vi "SID_filter_V2.vi"(5 "sampling info":cluster{"Fs":dbl, "#s":i32}={"Fs"=44100.0, "#s"=50}, 6 "reset":bool, 7 "filter":T1={"freq"=70.6, "res"=240.0, "HP"=FALSE, "BP"=FALSE, "LP"=TRUE, "VC1"=TRUE, "VC2"=TRUE, "VC3"=TRUE, "vol"=1.0} {"vol" format="%0.2f"; "res" format="%0.2f"; "freq" format="%0.2f"}, 9 "VC3":dbl[](array[numeric]), 10 "VC2":dbl[](array[numeric]), 11 "VC1":dbl[](array[numeric])) -> (3 "out":dbl[](array[numeric]))   [LabVIEW 2018]
uses:
  SID_filter_reg.ctl
panel:
  out "R":dbl
  out "Q":dbl
  out "g":dbl
  out "freq":dbl
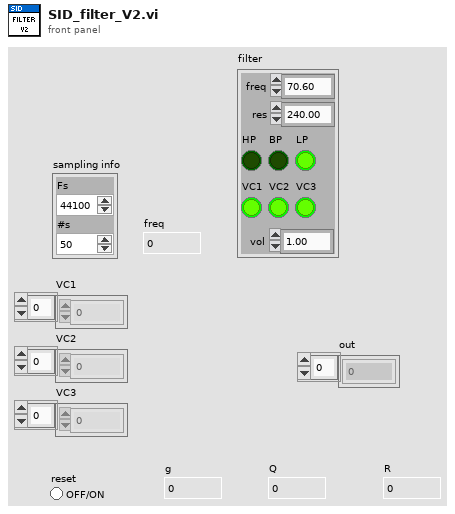
[diagram p1: front panel]
types:
  T1 = typedef "SID_filter_reg.ctl" = cluster{"freq":dbl, "res":dbl, "HP":bool, "BP":bool, "LP":bool, "VC1":bool, "VC2":bool, "VC3":bool, "vol":dbl}
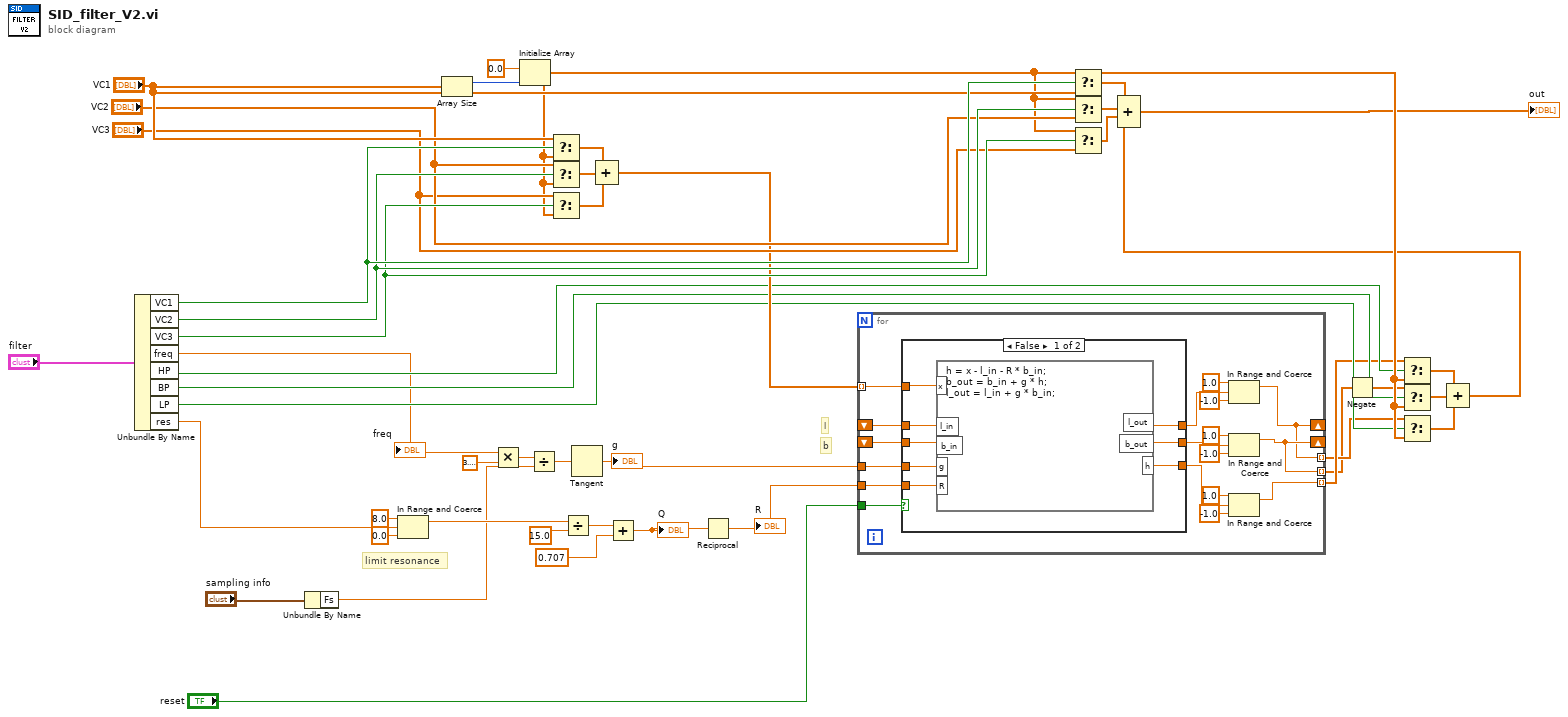
[diagram p0: block diagram]
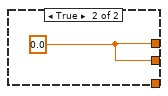
[diagram p2: hidden frame]
diagram:
  # "limit resonance"
  # "b"
  # "l"
  n1 = Unbundle By Name("filter") -> ("VC1"=w38:bool, "VC2"=w37:bool, "VC3"=w36:bool, "freq"=w4:dbl, "HP"=w17:bool, "BP"=w16:bool, "LP"=w15:bool, "res"=w11:dbl)
  "freq" <- w4
  n2 = Unbundle By Name("sampling info") -> ("Fs"=w8:dbl)
  n3 = In Range and Coerce(upper limit=8.0, x=w11, lower limit=0.0) -> (coerced(x)=w10:dbl)  [unwired: 1 out]
  n4 = Array Size(array="VC1") -> (size(s)=w46:i32)
  n5 = Multiply(x=w4, y=3.141592653589793) -> (x*y=w30:dbl)
  n6 = Initialize Array(0.0 ("element"), w46) -> (w18:dbl[])
  n7 = Divide(x=w30, y=w8) -> (x/y=w29:dbl)
  n8 = Select(t="VC1", s=w38, f=w18) -> (s? t:f=w44:dbl[])
  n9 = Select(t="VC2", s=w37, f=w18) -> (s? t:f=w43:dbl[])
  n10 = Select(t="VC3", s=w36, f=w18) -> (s? t:f=w42:dbl[])
  n11 = Divide(x=w10, y=15.0 ("Q")) -> (x/y=w27:dbl)
  n12 = Tangent(1:w29) -> (0:w23:dbl)
  "g" <- w23
  n13 = Compound Arithmetic op=ADD(w44, w43, w42) -> (w24:dbl[])
  n14 = Add(x=w27, y=0.707 ("Q")) -> (x+y=w25:dbl)
  "Q" <- w25
  n15 = Reciprocal(x=w25) -> (1/x=w22:dbl)
  "R" <- w22
  n16 = for {
    tunnel: w24 -> [w61] mode=indexing
    shift-right: [w51] -> _
    shift-left: _ -> [w63]
    shift-right: [w57] -> _
    shift-left: _ -> [w62]
    tunnel: "reset" -> [w64]
    tunnel: [w51] -> w6 mode=indexing
    tunnel: [w57] -> w2 mode=indexing
    tunnel: [w47] -> w14 mode=indexing
    tunnel: w23 -> [w60]
    tunnel: w22 -> [w59]
    n17 = case shown="False" w64 {
      tunnel: [w69 w73] -> w52
      tunnel: [w68 w73] -> w58
      tunnel: w63 -> [w71 _]
      tunnel: w62 -> [w70 _]
      tunnel: w61 -> [w72 _]
      tunnel: [w67 _] -> w48
      tunnel: w60 -> [w66 _]
      tunnel: w59 -> [w65 _]
      frame False {
        n18 = formula code="h = x - l_in - R * b_in;\nb_out = b_in + g * h;\nl_out = l_in + g * b_in;"("x"=w72, "l_in"=w71, "b_in"=w70, "g"=w66, "R"=w65) -> ("l_out"=w69:dbl, "b_out"=w68:dbl, "h"=w67:dbl)
      }
      frame True {
        w73 = 0.0 ("Q")
      }
    }
    n19 = In Range and Coerce(upper limit=1.0, x=w52, lower limit=-1.0) -> (coerced(x)=w51:dbl)  [unwired: 1 out]
    n20 = In Range and Coerce(upper limit=1.0, x=w58, lower limit=-1.0) -> (coerced(x)=w57:dbl)  [unwired: 1 out]
    n21 = In Range and Coerce(upper limit=1.0, x=w48, lower limit=-1.0) -> (coerced(x)=w47:dbl)  [unwired: 1 out]
  }
  n22 = Select(t=w18, s=w38, f="VC1") -> (s? t:f=w39:dbl[])
  n23 = Select(t=w18, s=w37, f="VC2") -> (s? t:f=w40:dbl[])
  n24 = Select(t=w18, s=w36, f="VC3") -> (s? t:f=w41:dbl[])
  n25 = Negate(x=w2) -> (-x=w1:dbl[])
  n26 = Select(t=w14, s=w17, f=w18) -> (s? t:f=w21:dbl[])
  n27 = Select(t=w1, s=w16, f=w18) -> (s? t:f=w20:dbl[])
  n28 = Select(t=w6, s=w15, f=w18) -> (s? t:f=w19:dbl[])
  n29 = Compound Arithmetic op=ADD(w21, w20, w19) -> (w5:dbl[])
  n30 = Compound Arithmetic op=ADD(w39, w40, w41, w5) -> (→"out":dbl[])
